vi "Total Shift.vi"(8 "error in (no error)":errorcluster, 11 "connection reference":T1) -> (0 "error out":errorcluster, 2 "Shift Hrs":i32)   [LabVIEW 2017]
uses:
  <vilib>/addons/database/Connection.llb/Conn ObjectReference.ctl
  <vilib>/addons/database/Connection.llb/Conn Execute.vi
  <vilib>/addons/database/Recordset.llb/Rec Fetch Recordset Data (R).vi
  <vilib>/addons/database/NI_Database_API.lvlib
panel:
  out "Total Shifts":i32
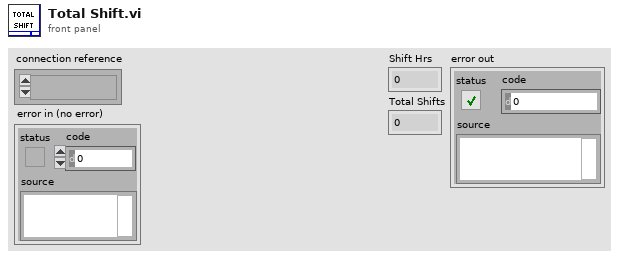
[diagram p1: front panel]
types:
  T1 = typedef "NI_Database_API.lvlib/Conn ObjectReference.ctl" = refnum<k1>
  T2 = typedef "NI_Database_API.lvlib/Rec ObjectReference.ctl" = refnum<k1>
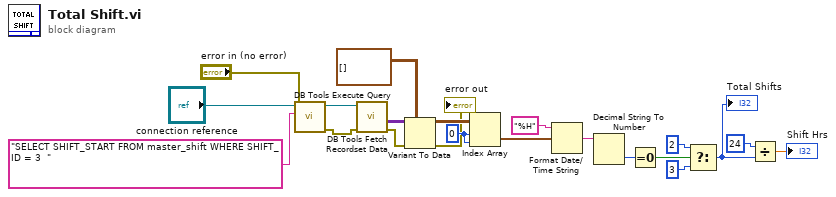
[diagram p0: block diagram]
diagram:
  w15 = 0 ("index (row)")
  n1 = call-poly <vilib>:"DB Tools Execute Query.vi"("error in (no error)"="error in (no error)", "SQL query"="SELECT SHIFT_START FROM master_shift WHERE SHIFT_ID = 3  ", "connection reference"="connection reference") -> ("error out"=w4:errorcluster, "recordset reference"=w20:T2)  [unwired: 5 in]
  n2 = call-poly <vilib>:"DB Tools Fetch Recordset Data.vi"("error in (no error)"=w4, "recordset reference"=w20) -> ("error out"=w3:errorcluster, "recordset data"=w19:variant[][])  [unwired: 3 in, 1 out]
  n3 = Variant To Data(error in=w3, type=timestamp[][] [] ("From Date 2"), Variant=w19) -> (data=w16:timestamp[][], error out=→"error out":errorcluster)
  n4 = Index Array(array=w16, index (row)=w15, index (col)=w15) -> (element=w14:timestamp)
  n5 = Format Date/Time String(time format string (%c)="%H", seconds (now)=w14) -> (date/time string=w9:string)  [unwired: 1 in]
  n6 = Decimal String To Number(string=w9) -> (number=w8:i32)  [unwired: 2 in, 1 out]
  n7 = Equal To 0?(x=w8) -> (x = 0?=w10:bool)
  n8 = Select(t=2, s=w10, f=3) -> (s? t:f=w7:i32)
  "Total Shifts" <- w7
  n9 = Divide(x=24, y=w7) -> (x/y=→"Shift Hrs":dbl)
